vi "Particle Filter.vi"() -> ()   [LabVIEW 2014]
doc: "This example performs a series of grayscale filtering, threshold, binary morphology, and particle analysis operations to measure the areas of all the large circular particles of the image."
uses:
  <vilib>/vision/NI_Vision_Development_Module.lvlib
panel:
  in  "Tab Control":T1(tab)
  out "Original":T2(plugin-control) caption="Original Image"
  out "Threshold":T2(plugin-control) caption="Threshold Image"
  out "Fill Hole and Reject Border":T2(plugin-control) caption="Reject Border and Fill Holes"
  out "Filter and Overlay Area":T2(plugin-control) caption="Filter Out Non Circles and Overlay Particle Area"
  # "Overview: Demonstrates how to use the IMAQ Particle Filter and other functions to remove unwanted particles from a binary image, and then IMAQ Particle Analysis is used to calculate the location and area of the remaining particles to overlay the results on the image. \nRequirements: Vision Development Software.\nInstructions: Run the VI, and click on the different tabs to see how the image is processed."
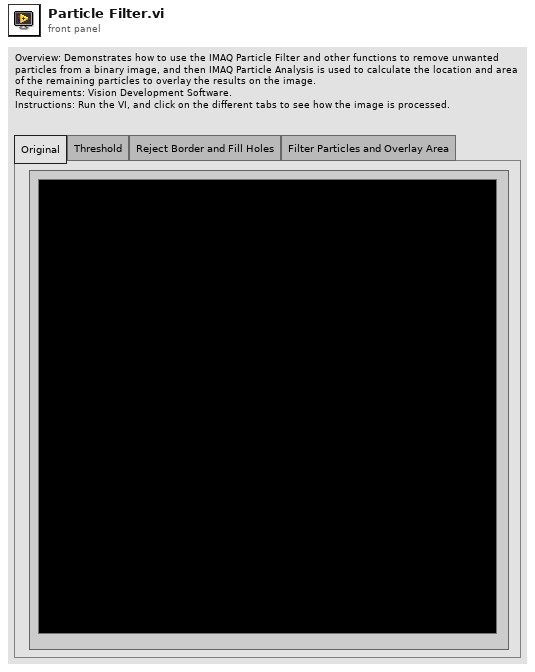
[diagram p1: front panel]
types:
  T1 = enum32{"Original", "Threshold", "Reject Border and Fill Holes", "Filter Particles and Overlay Area"}
  T2 = typedef "IMAQ Image.ctl" = refnum<image>
  T3 = typedef "Particle Parameters" = i32
  T4 = cluster{"Measurement Parameter":T3, "Range Lower Value":dbl, "Range Upper Value":dbl, "Range":bool, "Measurement Type":bool}[]
  T5 = cluster{"Desired Font (Application)":enum16{"User-specified Font", "Application Font", "System Font", "Dialog Font"}, "[User-specified Font]":cluster{"Font Name":string, "Size":i16, "Strikeout?":bool, "Italic?":bool, "Underline?":bool, "Outline?":bool, "Shadow?":bool, "Bold?":bool, "Rotation Angle":dbl}, "Horizontal Alignment":i16, "Vertical Alignment":i16}
  T6 = cluster{"Particle Measurements (Pixels)[0]":dbl, "Particle Measurements (Pixels)[1]":dbl, "Particle Measurements (Pixels)[2]":dbl}
  T7 = cluster{"Particle Measurements (Pixels)[0]":dbl, "Particle Measurements (Pixels)[1]":dbl}
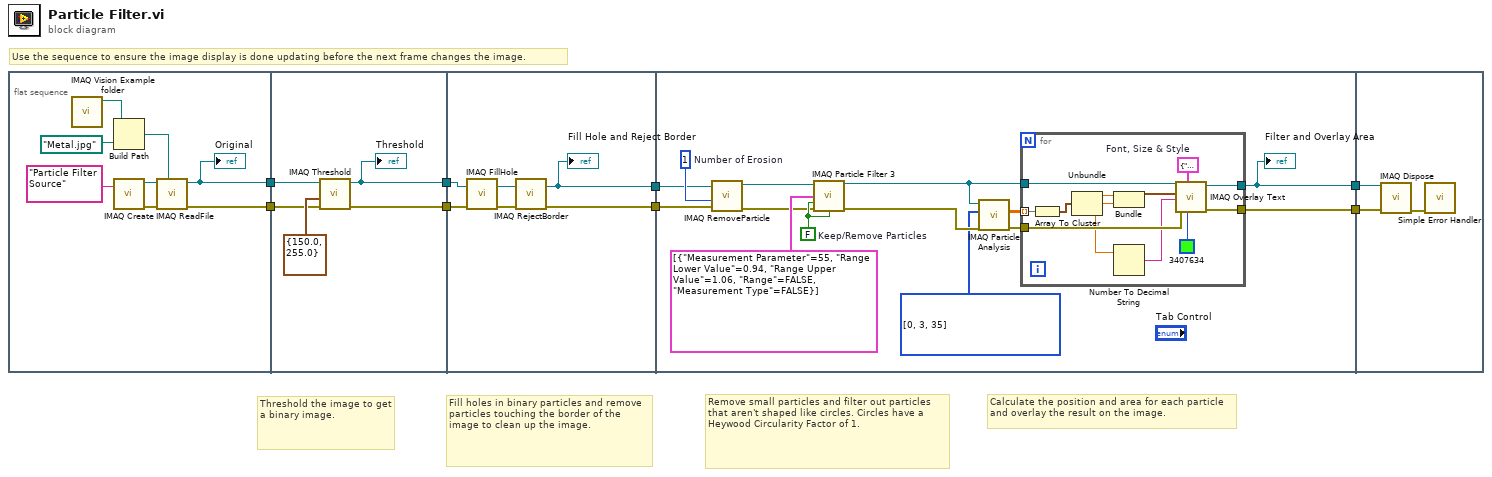
[diagram p0: block diagram]
diagram:
  # "Use the sequence to ensure the image display is done updating before the next frame changes the image."
  # "Calculate the position and area for each particle and overlay the result on the image."
  # "Remove small particles and filter out particles that aren't shaped like circles. Circles have a Heywood Circularity Factor of 1."
  # "Fill holes in binary particles and remove particles touching the border of the image to clean up the image."
  # "Threshold the image to get a binary image."
  n1 = flat-sequence {
    tunnel: [w10] -> w4
    tunnel: [w9] -> w3
    tunnel: [w19] -> w8
    tunnel: [w20] -> w7
    tunnel: w4 -> [w18]
    tunnel: w3 -> [w17]
    tunnel: w8 -> [w27]
    tunnel: w7 -> [w26]
    tunnel: [w22] -> w6
    tunnel: [w23] -> w5
    tunnel: w5 -> [w30]
    tunnel: w6 -> [w29]
    tunnel: [w36] -> w2
    tunnel: [w28] -> w1
    tunnel: w2 -> [w55]
    tunnel: w1 -> [w56]
    frame #0 {
      n2 = call "IMAQ Vision Example folder.vi"() -> ("Example Image Path"=w15:path)  [unwired: 11 in]
      n3 = Build Path(base path=w15, name or relative path=path "Metal.jpg") -> (appended path=w16:path)
      n4 = call "IMAQ Create"("Image Name"="Particle Filter Source") -> ("New Image"=w12:T2, "error out"=w11:errorcluster)  [unwired: 4 in]
      n5 = call "IMAQ ReadFile"("File Path"=w16, "error in (no error)"=w11, "Image"=w12) -> ("error out"=w9:errorcluster, "Image Out"=w10:T2)  [unwired: 4 in, 3 out]
      "Original" <- w10
    }
    frame #1 {
      n6 = call "IMAQ Threshold"("error in (no error)"=w17, "Range"=cluster{"Lower value":sgl, "Upper value":sgl} {"Lower value"=150.0, "Upper value"=255.0}, "Image Src"=w18) -> ("error out"=w20:errorcluster, "Image Dst Out"=w19:T2)  [unwired: 7 in]
      "Threshold" <- w19
    }
    frame #2 {
      n7 = call "IMAQ FillHole"("error in (no error)"=w26, "Image Src"=w27) -> ("error out"=w24:errorcluster, "Image Dst Out"=w25:T2)  [unwired: 4 in]
      n8 = call "IMAQ RejectBorder"("error in (no error)"=w24, "Image Src"=w25) -> ("error out"=w23:errorcluster, "Image Dst Out"=w22:T2)  [unwired: 4 in]
      "Fill Hole and Reject Border" <- w22
    }
    frame #3 {
      w33 = 1  # Number of Erosion
      w35 = FALSE  # Keep/Remove Particles
      w37 = T3[] [0, 3, 35] items=["Center of Mass X", "Center of Mass Y", "First Pixel X", "First Pixel Y", "Bounding Rect Left", "Bounding Rect Top", "Bounding Rect Right", "Bounding Rect Bottom", "Max Feret Diameter Start X", "Max Feret Diameter Start Y", "Max Feret Diameter End X", "Max Feret Diameter End Y", "Max Horiz. Segment Length Left", "Max Horiz. Segment Length Right", "Max Horiz. Segment Length Row", "-", "Bounding Rect Width", "Bounding Rect Height", "Bounding Rect Diagonal", "Perimeter", "Convex Hull Perimeter", "Holes' Perimeter", "Max Feret Diameter", "Equivalent Ellipse Major Axis", "Equivalent Ellipse Minor Axis", "Equivalent Ellipse Minor Axis (Feret)", "Equivalent Rect Long Side", "Equivalent Rect Short Side", "Equivalent Rect Diagonal", "Equivalent Rect Short Side (Feret)", "Average Horiz. Segment Length", "Average Vert. Segment Length", "Hydraulic Radius", "Waddel Disk Diameter", "-", "Area", "Holes' Area", "Particle & Holes' Area", "Convex Hull Area", "Image Area", "-", "Number of Holes", "Number of Horiz. Segments", "Number of Vert. Segments", "-", "Orientation", "Max Feret Diameter Orientation", "-", "% Area/Image Area", "% Area/(Particle & Holes' Area)", "Ratio of Equivalent Ellipse Axes", "Ratio of Equivalent Rect Sides", "-", "Elongation Factor", "Compactness Factor", "Heywood Circularity Factor", "Type Factor", "-", "Sum X", "Sum Y", "Sum XX", "Sum XY", "Sum YY", "Sum XXX", "Sum XXY", "Sum XYY", "Sum YYY", "-", "Moment of Inertia XX", "Moment of Inertia XY", "Moment of Inertia YY", "Moment of Inertia XXX", "Moment of Inertia XXY", "Moment of Inertia XYY", "Moment of Inertia YYY", "Norm. Moment of Inertia XX", "Norm. Moment of Inertia XY", "Norm. Moment of Inertia YY", "Norm. Moment of Inertia XXX", "Norm. Moment of Inertia XXY", "Norm. Moment of Inertia XYY", "Norm. Moment of Inertia YYY", "Hu Moment 1", "Hu Moment 2", "Hu Moment 3", "Hu Moment 4", "Hu Moment 5", "Hu Moment 6", "Hu Moment 7"] ("Pixel Measurements")
      n9 = call "IMAQ RemoveParticle"("error in (no error)"=w30, "Number of Erosion"=w33, "Image Src"=w29) -> ("error out"=w31:errorcluster, "Image Dst Out"=w32:T2)  [unwired: 7 in]
      n10 = call "IMAQ Particle Filter 3"("Image Src"=w32, "Selection Values"=T4 [{"Measurement Parameter"=55, "Range Lower Value"=0.94, "Range Upper Value"=1.06, "Range"=FALSE, "Measurement Type"=FALSE}], "Keep/Remove Particles (F)"=w35, "error in (no error)"=w31, "Fill Holes? (F)"=w35) -> ("Image Dst Out"=w40:T2, "error out"=w41:errorcluster)  [unwired: 8 in, 1 out]
      n11 = call "IMAQ Particle Analysis"("error in (no error)"=w41, "Pixel Measurements"=w37, "Image"=w40) -> ("error out"=w38:errorcluster, "Particle Measurements (Pixels)"=w39:dbl[][])  [unwired: 3 in, 4 out]
      n12 = for {
        tunnel: w38 -> [w54]
        tunnel: [w53] -> w36
        tunnel: [w52] -> w28
        tunnel: w40 -> [w49]
        tunnel: w39 -> [w43] mode=indexing
        w42 = T5 {"Desired Font (Application)"=enum."Application Font", "[User-specified Font]"={"Font Name"="", "Size"=12, "Strikeout?"=FALSE, "Italic?"=FALSE, "Underline?"=FALSE, "Outline?"=FALSE, "Shadow?"=FALSE, "Bold?"=FALSE, "Rotation Angle"=0.0}, "Horizontal Alignment"=0, "Vertical Alignment"=0}  # Font, Size & Style
        n13 = Array To Cluster(array=w43) -> (cluster=w48:T6)
        n14 = Unbundle(w48) -> ("Particle Measurements (Pixels)[0]"=w47:dbl, "Particle Measurements (Pixels)[1]"=w46:dbl, "Particle Measurements (Pixels)[2]"=w44:dbl)
        n15 = Bundle("Particle Measurements (Pixels)[0]"=w47, "Particle Measurements (Pixels)[1]"=w46) -> (w45:T7)  [unwired: 1 in]
        n16 = Number To Decimal String(number=w44) -> (decimal integer string=w51:string)  [unwired: 1 in]
        n17 = call "IMAQ Overlay Text"("Text Color (black)"=u32 3407634, "Font, Size & Style"=w42, "error in (no error)"=w54, "String"=w51, "Origin"=w45, "Image"=w49) -> ("error out"=w53:errorcluster, "Image Out"=w52:T2)  [unwired: 4 in]
      }
      "Filter and Overlay Area" <- w28
    }
    frame #4 {
      n18 = call "IMAQ Dispose"("Image"=w56, "error in (no error)"=w55) -> ("error out"=w57:errorcluster)  [unwired: 4 in]
      n19 = call <vilib>:"Simple Error Handler.vi"("error in (no error)"=w57) -> ()  [unwired: 4 in, 5 out]
    }
  }
